vi "DebCommandLog.vi"() -> ()   [LabVIEW 2018]
panel:
  in  "DebugLog":string[][](table)
  in  "DebugRun":bool
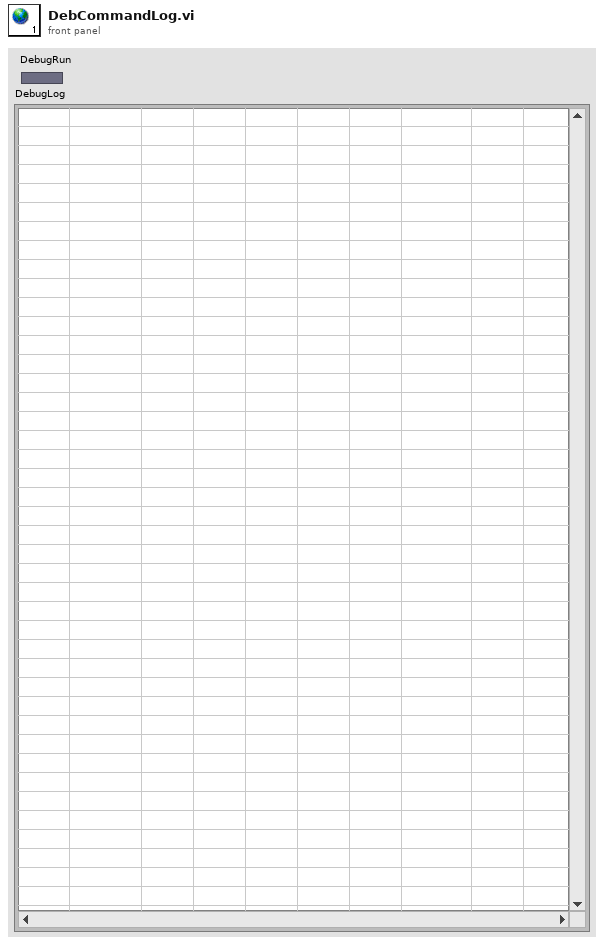
[diagram p1: front panel]
diagram:
